vi "AlliGator Compute & Plot All ROIs Characteristics.vi"(6 "ROI Statistics Selection":T1={"Area (pixels)"=TRUE, "% of Image"=TRUE, "Total Intensity"=TRUE, "Mean Intensity"=TRUE, "Median Intensity"=TRUE, "Mode Intensity"=TRUE, "Intensity Standard Deviation"=TRUE, "Min Intensity"=TRUE, "Max Intensity"=TRUE, "Mean SNR"=TRUE, "Median SNR"=TRUE, "Mode SNR"=TRUE, "SNR Standard Deviation"=TRUE, "Max SNR"=TRUE, "Min SNR"=TRUE, "# Rejected Pixels (NaN, Inf)"=TRUE, "# Negative Pixels"=TRUE, "Long Axis Length"=FALSE, "Short Axis Length"=FALSE, "Aspect Ratio"=FALSE}, 7 "Lifetime Graph":refnum<vi>, 8 "error in (no error)":errorcluster, 10 "ROI Mask Refnum":T3, 11 "Source Image Refnum":T3) -> (0 "error out":errorcluster, 1 "ROI Statistics String":string)   [LabVIEW 2021, in "AlliGator ROIs.lvlib"]
doc: "Computes all Source Image ROI characteristics and sends them as plots to the Lifetime & Other Parameters Graph."
uses:
  AlliGator ROIs.lvlib
  <vilib>/vision/Image Controls.llb/IMAQ Image.ctl
  Image/Image ROI Statistics.ctl
  Image/Image ROI Statistics Selection.ctl
  AlliGator Variables List.ctl
  Image/Named ROI Description.ctl
  AlliGator Globals, Variables & Constants.lvlib
  Image/Image.lvlib
  Graphs/XY Graph/XY Graph Add-Ons.lvlib
panel:
  out "ROI Statistics":T2
  # "see the AlliGator License on the block diagram (Ctrl+E or Window:Show Block Diagram)"
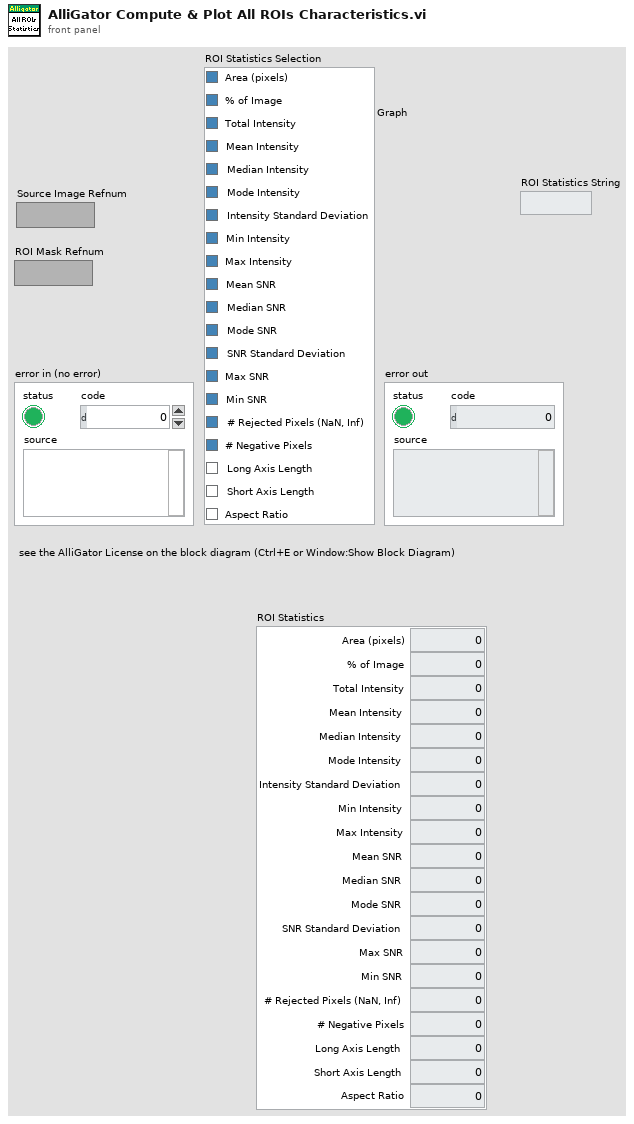
[diagram p1: front panel]
types:
  T1 = typedef "Image.lvlib/Image ROI Statistics Selection.ctl" = cluster{"Area (pixels)":bool, "% of Image":bool, "Total Intensity":bool, "Mean Intensity":bool, "Median Intensity":bool, "Mode Intensity":bool, "Intensity Standard Deviation":bool, "Min Intensity":bool, "Max Intensity":bool, "Mean SNR":bool, "Median SNR":bool, "Mode SNR":bool, "SNR Standard Deviation":bool, "Max SNR":bool, "Min SNR":bool, "# Rejected Pixels (NaN, Inf)":bool, "# Negative Pixels":bool, "Long Axis Length":bool, "Short Axis Length":bool, "Aspect Ratio":bool}
  T2 = typedef "Image.lvlib/Image ROI Statistics.ctl" = cluster{"Area (pixels)":dbl, "% of Image":dbl, "Total Intensity":dbl, "Mean Intensity":dbl, "Median Intensity":dbl, "Mode Intensity":dbl, "Intensity Standard Deviation":dbl, "Min Intensity":dbl, "Max Intensity":dbl, "Mean SNR":dbl, "Median SNR":dbl, "Mode SNR":dbl, "SNR Standard Deviation":dbl, "Max SNR":dbl, "Min SNR":dbl, "# Rejected Pixels (NaN, Inf)":dbl, "# Negative Pixels":dbl, "Long Axis Length":dbl, "Short Axis Length":dbl, "Aspect Ratio":dbl}
  T3 = typedef "IMAQ Image.ctl" = refnum<image>
  T4 = typedef "Image.lvlib/Named ROI Description.ctl" = cluster{"ROI Descriptor":T5, "ROI Name":string, "Overlay Color":u32}
  T5 = typedef "ROI Descriptor" = cluster{"Global Rectangle":i32[], "Contours":cluster{"ID":enum32{"External", "Internal"}, "Type":u32, "Coordinates":i32[]}[]}
  T6 = typedef "AlliGator Globals, Variables & Constants.lvlib/AlliGator Variables List.ctl" = enum16{"---- GUI ----", "GUI:Initialization Status", "GUI:State Indicators Refnum", "GUI:Original AlliGator Menu Items", "GUI:Current Action Loop State", "GUI:Script in progress", "GUI:Playback", "GUI:Loop Playback", "GUI:Search ROI Used", "GUI:Search ROI", "Decay Graph Max Legend Size", "Intensity Graph Max Legend Size", "Decay Statistics Graph Max Legend Size", "Phasor Graph Max Legend Size", "Phasor Ratio Graph Max Legend Size", "Lifetime Graph Max Legend Size", "---- Files ----", "Files:Export Dataset Frames as Individual Files", "Files:Show Batch Export Help Balloons", "Files:Frames in Dataset", "Files:ptu File Frame Start Indices", "Files:Current Frame in Dataset", "Files:Current Frame Timestamp", "Files:Dataset Loaded", "Files:Dataset Metadata", "Files:Dataset Channel", "Files:Dataset Data Description", "Files:Background Dataset Metadata", "Files:Background Dataset Channel", "Files:Background Dataset Data Description", "Files:Background File Subtraction", "Files:Background File Path", "Files:Background File Pile-up Correction", "Files:Background File Pixel Well Capacity", "Files:Background File Scaling Factor", "Files:Current Dataset Load Settings", "Files:Dataset Path", "Files:ICCD-specific Information", "Files:Macrotime Gate Separation", "------ Python Plugins ------", "Python Plugins:Information", "Python Plugins:Python Session", "Python Plugins:Valid Python Session?", "---- Source Image ----", "Source Image:ROIs", "Source Image:Current ROI", "Source Image:ROI Event Refnum", "X_Source Image Display Range", "X_Source Image Palette Information", "X_Type of Displayed Image", "X_Time Gate Slider", "Source Image:Palette List", "Source Image:Scale", "Source Image:ROI Overlay Color", "Source Image:Overlay to Erase", "Source Image:Is Displayed Image Accumulated", "---- Image Profile Window ----", "Image Profile:Overlay ROI in Source Image", "Image Profile:Window Event Refnum", "Image Profile:IntensityType", "Image Profile:Intensity Average Type", "Image Profile:Intensity-weighted SDV", "Image Profile:Box Profile Type", "Image Profile:Window Open", "Image Profile:Plotted Fit Parameter", "Source Image:White Light Image Modified", "Source Image:Mask Image Modified", "------ Phasor Graph -------", "Phasor Graph:Show Line", "---- Phasor Plot ---", "Phasor Plot Parameters Changed", "FLI Dataset Modified since last Phasor Plot Calculation", "Phasor Harmonics Data", "Selected Phasor Harmonics", "Phasor Harmonic Manager Event Refnum", "Phasor Plot ROIs", "Current Phasor Plot ROI", "Phasor Plot ROI Event Refnum", "Phasor Plot Image Reference Points", "Phasor Plot Computed", "Phasor Plot Palette Information", "Phasor Plot Palette List", "Phasor Ratio Palette Information", "Phasor Ratio Palette List", "Phasor Image Scale", "Phasor Plot Image Overlay to Erase", "Phasor Plot Image Elements to Update", "Current Phasor Plot Calculation Parameters", "Current Phasor Calibration Options", "Reset Cumulated Phasor Plot", "Phasor Ratio Reference 1", "Phasor Ratio Lifetime Reference 1", "Phasor Ratio Reference 1 Frequency", "Phasor Ratio Reference 2", "Phasor Ratio Lifetime Reference 2", "Phasor Ratio Reference 2 Frequency", "---- Decay Analysis ----", "Number of Selected Decays to Fit", "LS Fit Results", "LAR Fit Results", "BS Fit Results", "Last Decay Max - Min", "Best Fit Parameters", "Best Fit Parameter Names", "Actual Size X", "Actual Size Y", "Binning X", "Binning Y", "Actual # Gates", "Dataset Number", "Gates to...", "Gates Skipped", "Gates to keep", "Gate Step", "Gate Separation", "Reversed Gates", "Pile-up Correction", "Pixel Well Capacity", "Background Subtracted", "Background Subtraction Method", "Background Definition Range", "Background File (deprecated)", "Number of Dataset Accumulated", "Array of Accumulated Dataset Paths", "Do Averaged Datasets", "Destination File Path", "Process Plot Target", "Use 1/D as Phasor Frequency", "---- Decay Fit Parameter Map -----", "Decay Fit Parameter Map Palette Information", "Decay Fit Parameter Map Palette List", "Local Decay Graph Window Event Refnum", "------- Local Decay Window ---------", "Use normalized IRF for convolution", "----- Miscellaneous ----", "Skippable Dialog Windows Status"}
  T7 = typedef "XY Graph Add-Ons.lvlib/XY Graph Refnum.ctl" = refnum<vi>
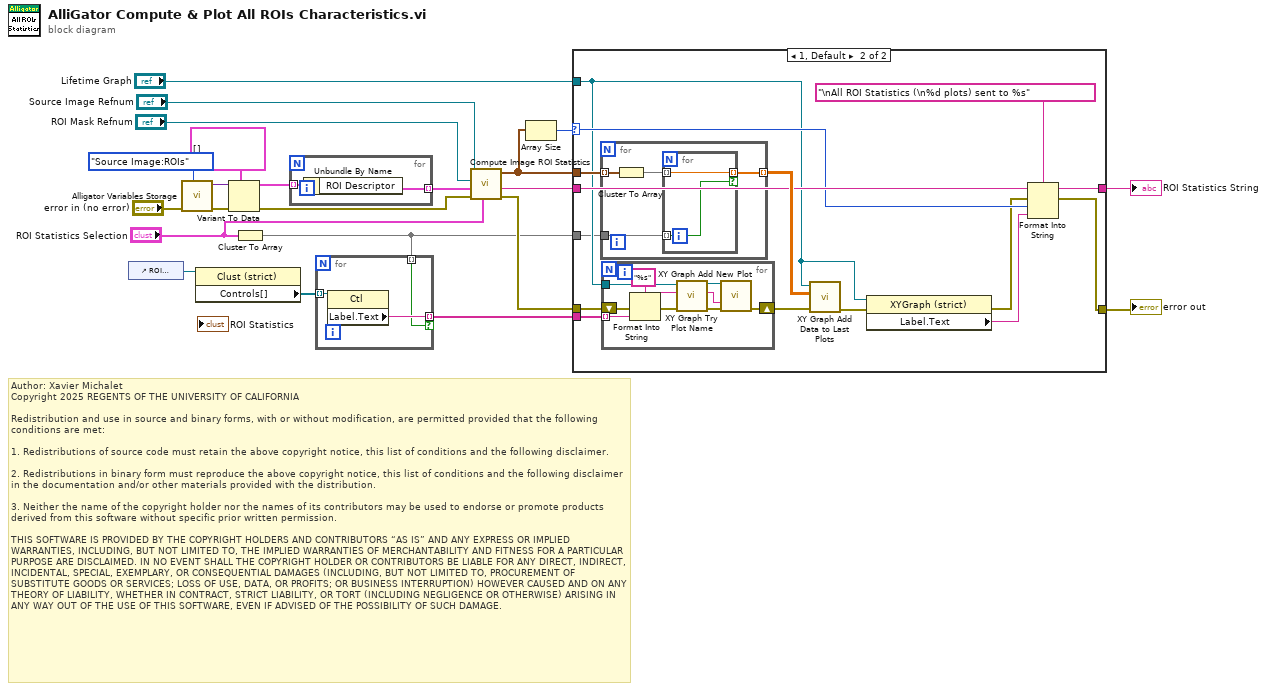
[diagram p0: block diagram]
diagram:
  # "Author: Xavier Michalet\nCopyright 2025 REGENTS OF THE UNIVERSITY OF CALIFORNIA\n\nRedistribution and use in source and binary forms, with or without modification, are permitted provided that the following conditions are met:\n\n1. Redistributions of source code must retain the above copyright notice, this list of conditions and the following disclaimer.\n\n2. Redistributions in binary form must reproduce the above copyright notice, this list of conditions and the following disclaimer in the documentation and/or other materials provided with the distribution.\n\n3. Neither the name of the copyright holder nor the names of its contributors may be used to endorse or promote products derived from this software without specific prior written permission.\n\nTHIS SOFTWARE IS PROVIDED BY THE COPYRIGHT HOLDERS AND CONTRIBUTORS “AS IS” AND ANY EXPRESS OR IMPLIED WARRANTIES, INCLUDING, BUT NOT LIMITED TO, THE IMPLIED WARRANTIES OF MERCHANTABILITY AND FITNESS FOR A PARTICULAR PURPOSE ARE DISCLAIMED. IN NO EVENT SHALL THE COPYRIGHT HOLDER OR CONTRIBUTORS BE LIABLE FOR ANY DIRECT, INDIRECT, INCIDENTAL, SPECIAL, EXEMPLARY, OR CONSEQUENTIAL DAMAGES (INCLUDING, BUT NOT LIMITED TO, PROCUREMENT OF SUBSTITUTE GOODS OR SERVICES; LOSS OF USE, DATA, OR PROFITS; OR BUSINESS INTERRUPTION) HOWEVER CAUSED AND ON ANY THEORY OF LIABILITY, WHETHER IN CONTRACT, STRICT LIABILITY, OR TORT (INCLUDING NEGLIGENCE OR OTHERWISE) ARISING IN ANY WAY OUT OF THE USE OF THIS SOFTWARE, EVEN IF ADVISED OF THE POSSIBILITY OF SUCH DAMAGE."
  n1 = control-ref of="ROI Statistics"() -> (w11:refnum<vi>)
  n2 = call "Alligator Variables Storage.vi"("AlliGator Variable"=AlliGator_Variables_List."Source Image:ROIs" ("Alligator Variable"), "Error In"="error in (no error)") -> ("Error Out"=w15:errorcluster, "Data out"=w14:variant)  [unwired: 7 in, 1 out]
  n3 = property class="Clust (strict)"(reference=w11) -> ("Controls[]"=w10:refnum<vi>[])  [unwired: 1 in, 2 out]
  n4 = Variant To Data(error in=w15, type=T4[] [] ("Stored ROIs in"), Variant=w14) -> (data=w19:T4[], error out=w18:errorcluster)
  n5 = Cluster To Array(cluster="ROI Statistics Selection") -> (array=w1:bool[])
  n6 = for {
    tunnel: w19 -> [w24] mode=indexing
    tunnel: [w23] -> w20 mode=indexing
    n7 = Unbundle By Name(w24) -> ("ROI Descriptor"=w23:T5)
  }
  n8 = for {
    tunnel: w10 -> [w27] mode=indexing
    tunnel: [w26] -> w9 mode=indexing if=w25
    tunnel: w1 -> [w25] mode=indexing
    n9 = property class="Ctl"(reference=w27) -> ("Label.Text"=w26:string)  [unwired: 1 in, 2 out]
  }
  n10 = call "Compute Image ROI Statistics.vi"("ROI Characteristics Selection"="ROI Statistics Selection", "error in (no error)"=w18, "ROIs"=w20, "ROI Mask Refnum"="ROI Mask Refnum", "Image Refnum"="Source Image Refnum") -> ("error out"=w12:errorcluster, "ROI Characteristics String"=w4:string, "ROI Characteristics"=w7:T2[])  [unwired: 4 in]
  n11 = Array Size(array=w7) -> (size(s)=w8:i32)
  n12 = case shown="1, Default" w8 {
    selector: w8 -> [_ w36]
    tunnel: w12 -> [w29 w44]
    tunnel: w9 -> [_ w43]
    tunnel: w7 -> [_ w41]
    tunnel: "Lifetime Graph" -> [_ w31]
    tunnel: [w29 w37] -> w5
    tunnel: w4 -> [w28 w39]
    tunnel: [w28 w38] -> w3
    tunnel: w1 -> [_ w30]
    frame 0 {
    }
    frame 1, Default {
      n13 = for {
        tunnel: w41 -> [w48] mode=indexing
        tunnel: [w45] -> w40 mode=indexing
        tunnel: w30 -> [w46]
        n14 = Cluster To Array(cluster=w48) -> (array=w47:dbl[])
        n15 = for {
          tunnel: w47 -> [w50] mode=indexing
          tunnel: w46 -> [w49] mode=indexing
          tunnel: [w50] -> w45 mode=indexing if=w49
        }
      }
      n16 = for {
        shift-right: [w59] -> w42
        shift-left: w44 -> [w56]
        tunnel: w43 -> [w52] mode=indexing
        tunnel: w31 -> [w51]
        n17 = Format Into String(format string="%s", error in=w56, w52) -> (resulting string=w54:string, error out=w55:errorcluster)  [unwired: 1 in]
        n18 = call "XY Graph Try Plot Name.vi"("Error In"=w55, "Plot Name in"=w54, "XY Graph Refnum"=w51) -> ("Error Out"=w58:errorcluster, "Plot Name out"=w60:string, "XY Graph Refnum"=w53:T7)  [unwired: 5 in, 1 out]
        n19 = call "XY Graph Add New Plot.vi"("Multiplot XY Graph"=w53, "New Plot Name in"=w60, "error in (no error)"=w58) -> ("error out"=w59:errorcluster)  [unwired: 9 in, 3 out]
      }
      n20 = call "XY Graph Add Data to Last Plots.vi"("error in (no error)"=w42, "Plots Data Array"=w40, "XYGraph in"=w31) -> ("error out"=w34:errorcluster)  [unwired: 8 in]
      n21 = property class="XYGraph (strict)"(reference=w31, error in=w34) -> (error out=w33:errorcluster, "Label.Text"=w32:string)  [unwired: 1 out]
      n22 = Format Into String(format string="\nAll ROI Statistics (\n%d plots) sent to %s", initial string=w39, error in=w33, w36, w32) -> (resulting string=w38:string, error out=w37:errorcluster)
    }
  }
  "ROI Statistics String" <- w3
  "error out" <- w5
